vi "Accel self test.vi"(8 "error in (no error)":errorcluster, 11 "Accelerometer":T1) -> (0 "error out":errorcluster, 2 "accel self test":dbl[](array[numeric]), 3 "Accelerometer out":T1)   [LabVIEW 2013]
doc: "Use this template to build a VI to use as a subVI."
uses:
  AccelerometerSPI.ctl
  <vilib>/ni845x/ni845x.llb/ni845xControl.ctl
  <vilib>/ni845x/ni845x.llb/ni845xSpiConfiguration.ctl
  9250registers.ctl
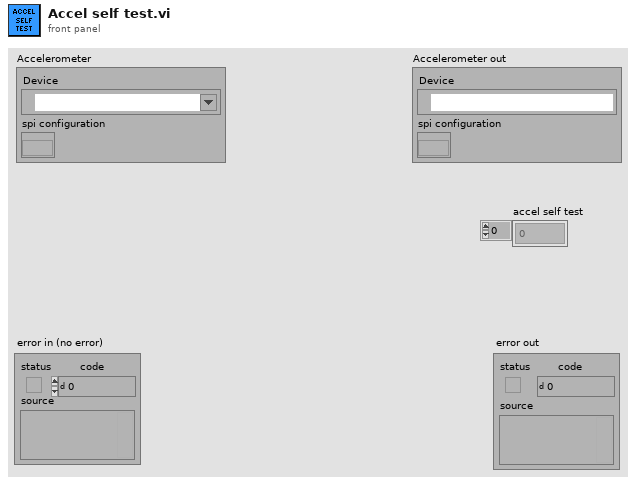
[diagram p1: front panel]
types:
  T1 = typedef "AccelerometerSPI.ctl" = cluster{"Device":T2, "spi configuration":T3}
  T2 = typedef "ni845xControl.ctl" = refnum<k21>
  T3 = typedef "ni845xSpiConfiguration.ctl" = refnum<k20>
  T4 = typedef "9250registers.ctl" = u8
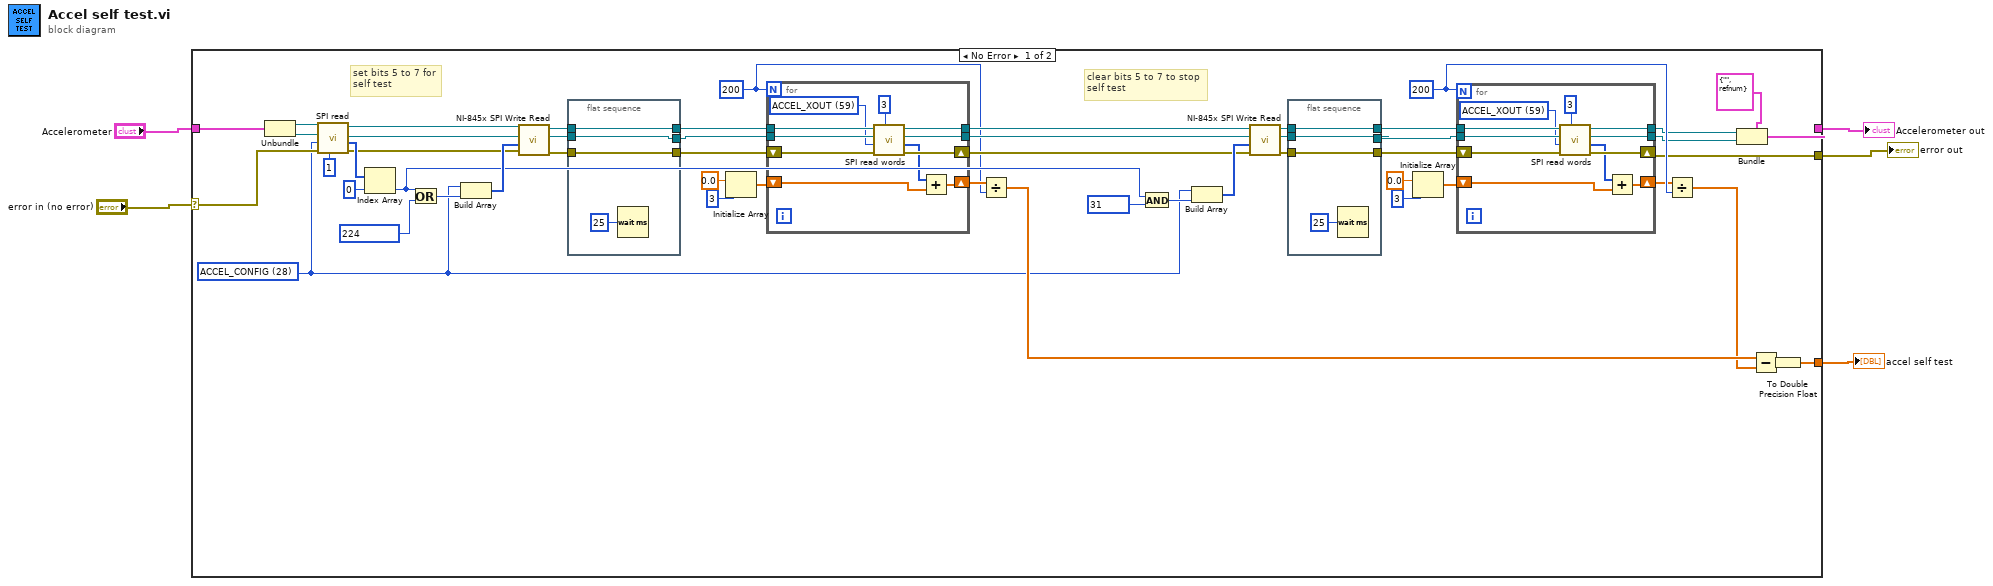
[diagram p0: block diagram]
diagram:
  n1 = case shown="No Error" "error in (no error)" {
    selector: "error in (no error)" -> [w54 w89]
    tunnel: [w7 w89] -> w2
    tunnel: "Accelerometer" -> [w57 w88]
    tunnel: [w38 w88] -> w3
    tunnel: [w37 _] -> w1
    frame No Error {
      w6 = T4 28 items=["SELF_TEST_X_GYRO"=0, "SELF_TEST_Y_GYRO"=1, "SELF_TEST_Z_GYRO"=2, "SELF_TEST_X_ACCEL"=13, "SELF_TEST_Y_ACCEL"=14, "SELF_TEST_Z_ACCEL"=15, "XG_OFFSET"=19, "YG_OFFSET"=21, "ZG_OFFSET"=23, "SMPLRT_DIV"=25, "CONFIG"=26, "GYRO_CONFIG"=27, "ACCEL_CONFIG"=28, "ACCEL_CONFIG2"=29, "FIFO_EN"=35, "I2C_MST_CTRL"=36, "I2C_SLV0_ADDR"=37, "I2C_SLV0_REG"=38, "I2C_SLV0_CTRL"=39, "I2C_MST_STATUS"=54, "INT_ENABLE"=56, "INT_STATUS"=58, "ACCEL_XOUT"=59, "ACCEL_YOUT"=61, "ACCEL_ZOUT"=63, "TEMP_OUT"=65, "GYRO_XOUT"=67, "GYRO_YOUT"=69, "GYRO_ZOUT"=71, "EXT_SENS_DATA_00"=73, "I2C_SLV0_D0"=99, "USER_CTRL"=106, "PWR_MGMT_1"=107, "PWR_MGMT_2"=108, "WHO_AM_I"=117, "XA_OFFSET"=119, "YA_OFFSET"=122, "ZA_OFFSET"=125] ("9250 Registers")
      w30 = 200
      w31 = 200
      # "clear bits 5 to 7 to stop\nself test"
      # "set bits 5 to 7 for\nself test"
      n2 = Unbundle(w57) -> ("Device"=w56:T2, "spi configuration"=w55:T3)
      n3 = call "SPI read.vi"("Number of bytes"=1, "error in (no error)"=w54, "Address"=w6, "spi configuration in"=w55, "Device ref in"=w56) -> ("error out"=w45:errorcluster, "read data"=w52:u8[], "spi configuration out"=w47:T3, "Device ref out"=w48:T2)  [unwired: 3 in]
      n4 = Index Array(array=w52, index=0) -> (element=w33:u8)
      n5 = Or(x=w33, y=u8 224) -> (x .or. y?=w49:u8)
      n6 = Build Array(w6, w49) -> (w46:T4[])
      n7 = call <vilib>:"NI-845x SPI Write Read.vi"("error in (no error)"=w45, "write data"=w46, "spi configuration in"=w47, "device reference in"=w48) -> ("error out"=w20:errorcluster, "spi configuration out"=w21:T3, "device reference out"=w22:T2)  [unwired: 4 in, 1 out]
      n8 = flat-sequence {
        tunnel: w22 -> [w64]
        tunnel: w21 -> [w63]
        tunnel: w20 -> [w62]
        tunnel: [w64] -> w19
        tunnel: [w63] -> w18
        tunnel: [w62] -> w17
        frame #0 {
          n9 = Wait (ms)(milliseconds to wait=u32 25) -> ()  [unwired: 1 out]
        }
      }
      n10 = Initialize Array(0.0 ("element"), 3 ("dimension size")) -> (w26:dbl[])
      n11 = for {
        N: w31 -> [_]
        tunnel: w19 -> [w87]
        tunnel: w18 -> [w86]
        tunnel: [w84] -> w36
        tunnel: [w83] -> w35
        shift-right: [w82] -> w34
        shift-left: w17 -> [w85]
        shift-right: [w78] -> w41
        shift-left: w26 -> [w80]
        w77 = T4 59 items=["SELF_TEST_X_GYRO"=0, "SELF_TEST_Y_GYRO"=1, "SELF_TEST_Z_GYRO"=2, "SELF_TEST_X_ACCEL"=13, "SELF_TEST_Y_ACCEL"=14, "SELF_TEST_Z_ACCEL"=15, "XG_OFFSET"=19, "YG_OFFSET"=21, "ZG_OFFSET"=23, "SMPLRT_DIV"=25, "CONFIG"=26, "GYRO_CONFIG"=27, "ACCEL_CONFIG"=28, "ACCEL_CONFIG2"=29, "FIFO_EN"=35, "I2C_MST_CTRL"=36, "I2C_SLV0_ADDR"=37, "I2C_SLV0_REG"=38, "I2C_SLV0_CTRL"=39, "I2C_MST_STATUS"=54, "INT_ENABLE"=56, "INT_STATUS"=58, "ACCEL_XOUT"=59, "ACCEL_YOUT"=61, "ACCEL_ZOUT"=63, "TEMP_OUT"=65, "GYRO_XOUT"=67, "GYRO_YOUT"=69, "GYRO_ZOUT"=71, "EXT_SENS_DATA_00"=73, "I2C_SLV0_D0"=99, "USER_CTRL"=106, "PWR_MGMT_1"=107, "PWR_MGMT_2"=108, "WHO_AM_I"=117, "XA_OFFSET"=119, "YA_OFFSET"=122, "ZA_OFFSET"=125] ("9250 Registers")
        n12 = call "SPI read words.vi"("Number of words"=3, "error in (no error)"=w85, "address"=w77, "spi configuration in"=w86, "Refnum in"=w87) -> ("error out"=w82:errorcluster, "data out"=w79:i16[], "spi configuration out"=w83:T3, "Refnum out"=w84:T2)  [unwired: 3 in]
        n13 = Add(x=w79, y=w80) -> (x+y=w78:dbl[])
      }
      n14 = Divide(x=w41, y=w31) -> (x/y=w32:dbl[])
      n15 = And(x=w33, y=u8 31) -> (x .and. y?=w43:u8)
      n16 = Build Array(w6, w43) -> (w44:T4[])
      n17 = call <vilib>:"NI-845x SPI Write Read.vi"("error in (no error)"=w34, "write data"=w44, "spi configuration in"=w35, "device reference in"=w36) -> ("error out"=w14:errorcluster, "spi configuration out"=w15:T3, "device reference out"=w16:T2)  [unwired: 4 in, 1 out]
      n18 = flat-sequence {
        tunnel: w16 -> [w60]
        tunnel: w15 -> [w59]
        tunnel: w14 -> [w58]
        tunnel: [w60] -> w13
        tunnel: [w59] -> w12
        tunnel: [w58] -> w11
        frame #0 {
          n19 = Wait (ms)(milliseconds to wait=u32 25) -> ()  [unwired: 1 out]
        }
      }
      n20 = Initialize Array(0.0 ("element"), 3 ("dimension size")) -> (w24:dbl[])
      n21 = for {
        N: w30 -> [_]
        tunnel: w13 -> [w76]
        tunnel: w12 -> [w75]
        tunnel: [w73] -> w9
        tunnel: [w72] -> w8
        shift-right: [w71] -> w7
        shift-left: w11 -> [w74]
        shift-right: [w67] -> w29
        shift-left: w24 -> [w69]
        w66 = T4 59 items=["SELF_TEST_X_GYRO"=0, "SELF_TEST_Y_GYRO"=1, "SELF_TEST_Z_GYRO"=2, "SELF_TEST_X_ACCEL"=13, "SELF_TEST_Y_ACCEL"=14, "SELF_TEST_Z_ACCEL"=15, "XG_OFFSET"=19, "YG_OFFSET"=21, "ZG_OFFSET"=23, "SMPLRT_DIV"=25, "CONFIG"=26, "GYRO_CONFIG"=27, "ACCEL_CONFIG"=28, "ACCEL_CONFIG2"=29, "FIFO_EN"=35, "I2C_MST_CTRL"=36, "I2C_SLV0_ADDR"=37, "I2C_SLV0_REG"=38, "I2C_SLV0_CTRL"=39, "I2C_MST_STATUS"=54, "INT_ENABLE"=56, "INT_STATUS"=58, "ACCEL_XOUT"=59, "ACCEL_YOUT"=61, "ACCEL_ZOUT"=63, "TEMP_OUT"=65, "GYRO_XOUT"=67, "GYRO_YOUT"=69, "GYRO_ZOUT"=71, "EXT_SENS_DATA_00"=73, "I2C_SLV0_D0"=99, "USER_CTRL"=106, "PWR_MGMT_1"=107, "PWR_MGMT_2"=108, "WHO_AM_I"=117, "XA_OFFSET"=119, "YA_OFFSET"=122, "ZA_OFFSET"=125] ("9250 Registers")
        n22 = call "SPI read words.vi"("Number of words"=3, "error in (no error)"=w74, "address"=w66, "spi configuration in"=w75, "Refnum in"=w76) -> ("error out"=w71:errorcluster, "data out"=w68:i16[], "spi configuration out"=w72:T3, "Refnum out"=w73:T2)  [unwired: 3 in]
        n23 = Add(x=w68, y=w69) -> (x+y=w67:dbl[])
      }
      n24 = Divide(x=w29, y=w30) -> (x/y=w10:dbl[])
      n25 = Bundle(cluster=T1 {"Device"="", "spi configuration"=refnum} ("Accelerometer"), "Device"=w9, "spi configuration"=w8) -> (w38:T1)
      n26 = Subtract(x=w32, y=w10) -> (x-y=w40:dbl[])
      n27 = To Double Precision Float(number=w40) -> (double precision float=w37:dbl[])
    }
    frame Error {
    }
  }
  "error out" <- w2
  "Accelerometer out" <- w3
  "accel self test" <- w1
